vi "Barcode Scan State.vi"(1 "Barcode Scan Refnum":refnum<vi>, 2 "Stop Button Ref":refnum<vi>, 5 "Queue in":refnum<queue>, 9 "Test Results":T1, 11 "error in (no error)":errorcluster) -> (8 "Number of Buttons":u32=14, 10 "Test Results Out":T1, 15 "error out":errorcluster)   [LabVIEW 2016]
doc: "This VI performs the Wait for Barcode Scan State. It reads the config file in a while loop until a valid model number is read. Then determines hardware type, and updates UI based on hardware type."
uses:
  controls/Test Results.ctl
  C:/Program Files (x86)/National Instruments/LabVIEW 2016/examples/Design Patterns/Queued Message Handler/support/QMH Fundamentals - Message Cluster.ctl
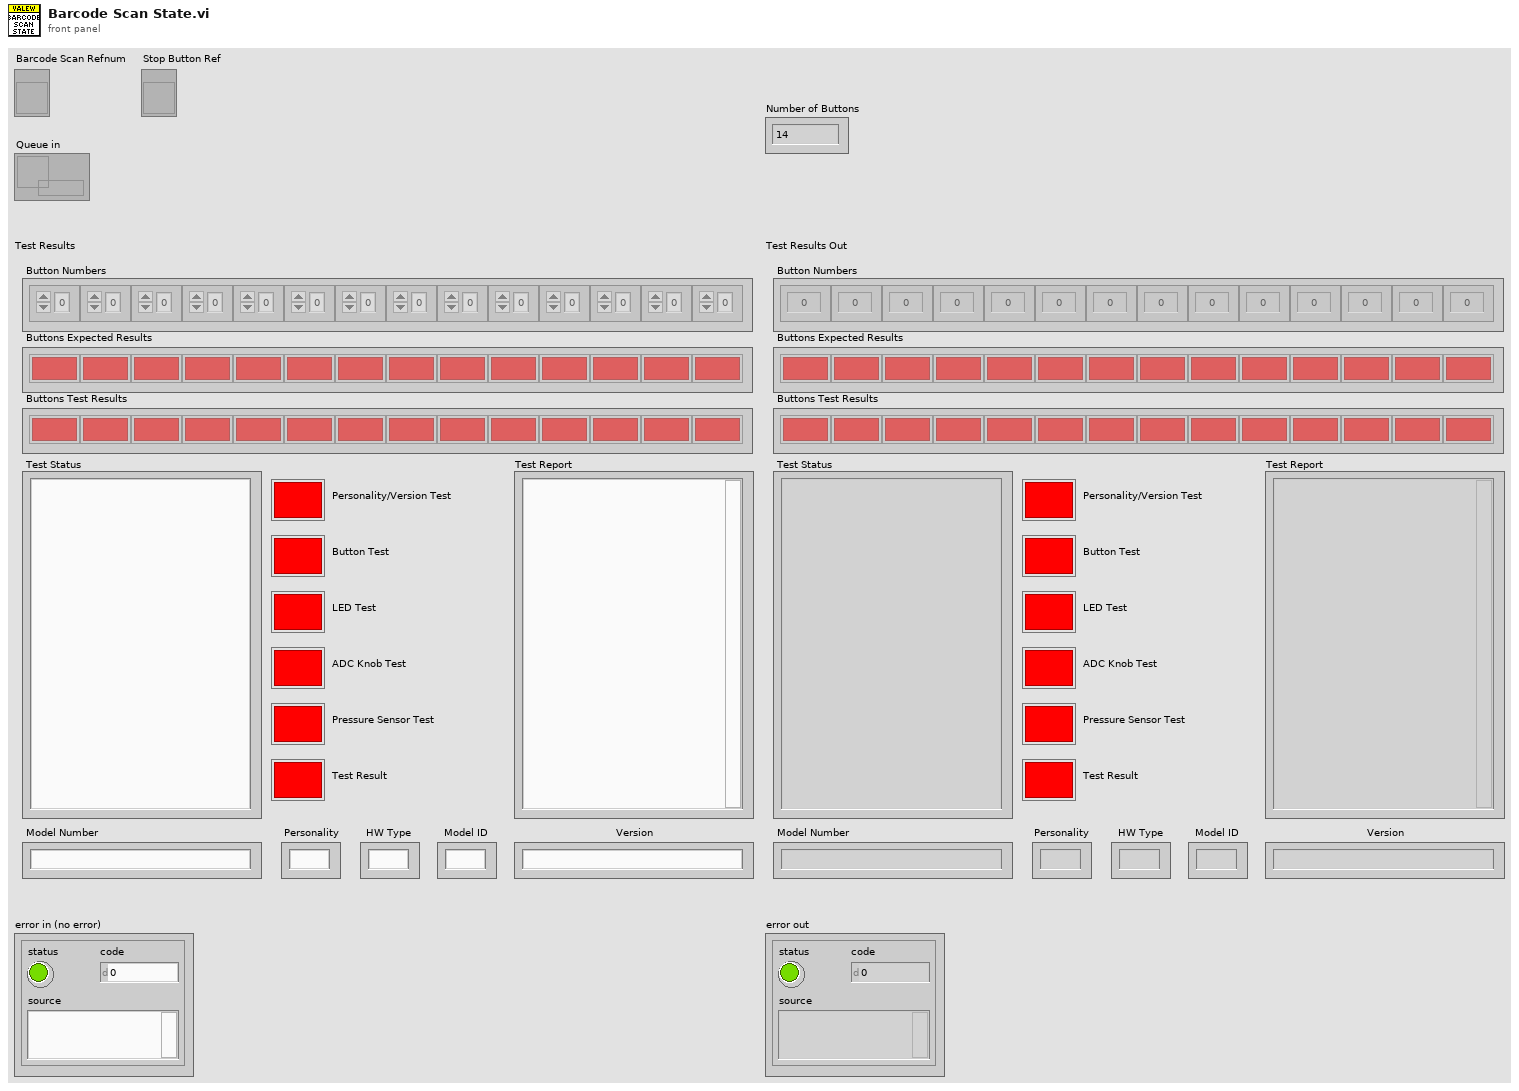
[diagram p1: front panel]
types:
  T1 = typedef "Test Results.ctl" = cluster{"Test Status":string, "Personality/Version Test ":bool, "Test Report":string, "Model Number":string, "Button Numbers":i32[], "Buttons Test Results":bool[], "Buttons Expected Results":bool[], "Model ID":string, "Personality":string, "HW Type":string, "Version":string, "Button Test":bool, "LED Test":bool, "ADC Knob Test":bool, "Pressure Sensor Test":bool, "Test Result":bool}
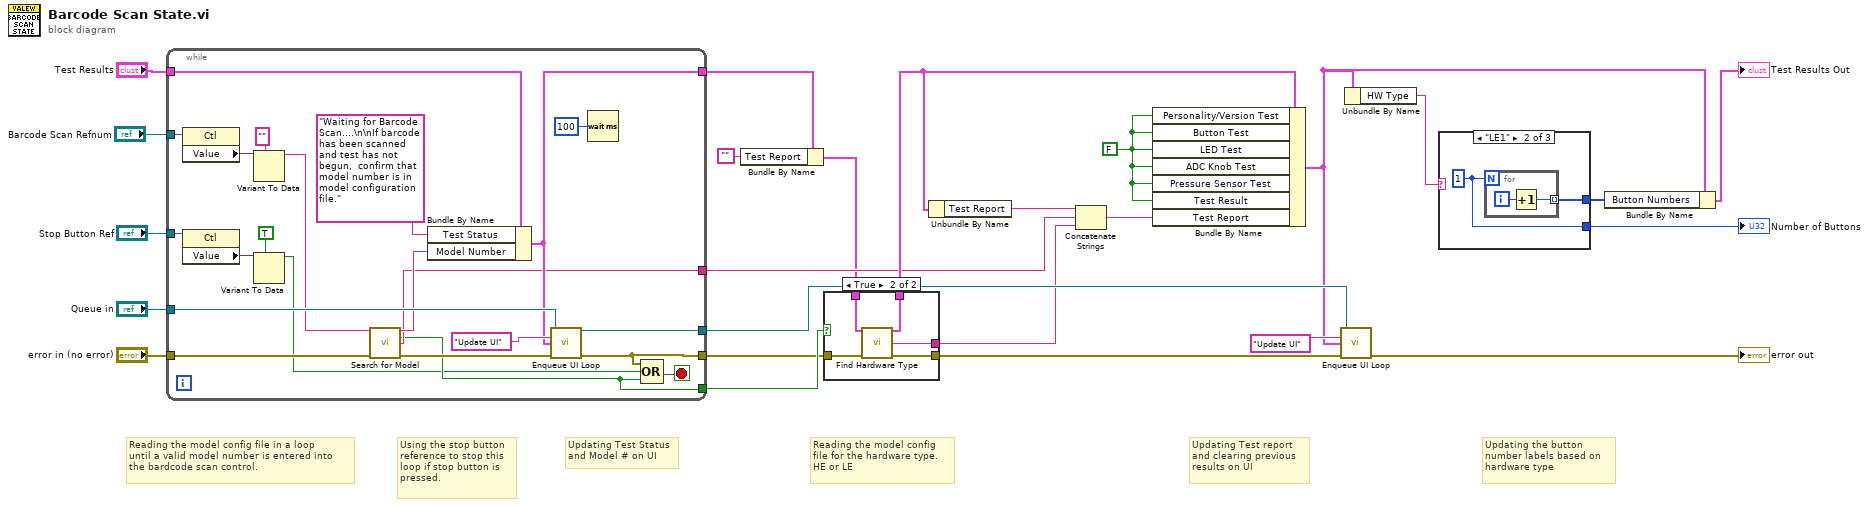
[diagram p0: block diagram]
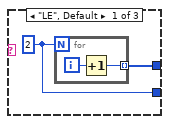
[diagram p2: hidden frame]
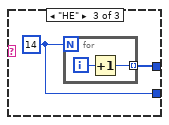
[diagram p3: hidden frame]
diagram:
  w1 = FALSE
  # "Updating Test Status\nand Model # on UI"
  # "Updating the button \nnumber labels based on \nhardware type"
  # "Updating Test report\nand clearing previous \nresults on UI"
  # "Reading the model config \nfile for the hardware type.\nHE or LE"
  # "Reading the model config file in a loop\nuntil a valid model number is entered into \nthe bardcode scan control."
  # "Using the stop button\nreference to stop this \nloop if stop button is\npressed."
  n1 = while {
    tunnel: "Test Results" -> [w44]
    tunnel: "error in (no error)" -> [w46]
    tunnel: "Queue in" -> [w41]
    tunnel: [w39] -> w5
    tunnel: [w35] -> w20
    tunnel: [w37] -> w22
    tunnel: [w36] -> w12
    tunnel: [w34] -> w25
    tunnel: "Barcode Scan Refnum" -> [w33]
    tunnel: "Stop Button Ref" -> [w28]
    stop <- w45 stop-if-true
    n2 = property class="Ctl"(reference=w33) -> ("Value"=w32:variant)  [unwired: 1 in, 2 out]
    n3 = property class="Ctl"(reference=w28) -> ("Value"=w29:variant)  [unwired: 1 in, 2 out]
    n4 = Variant To Data(type="", Variant=w32) -> (data=w31:string)  [unwired: 1 in, 1 out]
    n5 = Variant To Data(type=TRUE, Variant=w29) -> (data=w27:bool)  [unwired: 1 in, 1 out]
    n6 = call "Search for Model.vi"("Barcode Scan"=w31, "error in (no error)"=w46) -> ("Model Number"=w38:string, "Model Found?"=w34:bool, "Report Text"=w36:string, "error out"=w42:errorcluster)  [unwired: 10 in]
    n7 = Bundle By Name(cluster=w44, "Test Status"="Waiting for Barcode Scan....\n\nIf barcode has been scanned and test has not begun,  confirm that model number is in model configuration file.", "Model Number"=w38) -> (w39:T1)
    n8 = call "Enqueue UI Loop.vi"("UI Que In"=w41, "Message"="Update UI", "Test Results"=w39, "error in (no error)"=w42) -> ("UI Queue Out"=w37:refnum<queue>, "error out"=w35:errorcluster)  [unwired: 10 in]
    n9 = Wait (ms)(milliseconds to wait=u32 100) -> ()  [unwired: 1 out]
    n10 = Compound Arithmetic op=OR(w35, w27, w34) -> (w45:bool)
  }
  n11 = Bundle By Name(cluster=w5, "Test Report"="") -> (w4:T1)
  n12 = case shown="True" w25 {
    tunnel: w20 -> [w48 w54]
    tunnel: [w48 w53] -> w24
    tunnel: w4 -> [w49 w52]
    tunnel: [w49 w51] -> w13
    tunnel: [_ w50] -> w10
    frame False {
    }
    frame True {
      n13 = call "Find Hardware Type.vi"("Test Results In"=w52, "error in (no error)"=w54) -> ("Test Results Out"=w51:T1, "Report Text"=w50:string, "error out"=w53:errorcluster)  [unwired: 10 in, 1 out]
    }
  }
  n14 = Unbundle By Name(w13) -> ("Test Report"=w14:string)
  n15 = Concatenate Strings(w14, w12, w10) -> (w11:string)
  n16 = Bundle By Name(cluster=w13, "Personality/Version Test"=w1, "Button Test"=w1, "LED Test"=w1, "ADC Knob Test"=w1, "Pressure Sensor Test"=w1, "Test Result"=w1, "Test Report"=w11) -> (w8:T1)
  n17 = call "Enqueue UI Loop.vi"("UI Que In"=w22, "Message"="Update UI", "Test Results"=w8, "error in (no error)"=w24) -> ("error out"=→"error out":errorcluster)  [unwired: 10 in, 1 out]
  n18 = Unbundle By Name(w8) -> ("HW Type"=w9:string)
  n19 = case shown="\"LE1\"" w9 {
    tunnel: [w56 w60 w64] -> w7
    tunnel: [w55 w59 w63] -> w2
    frame "LE", Default {
      w55 = u32 2
      n20 = for {
        N: w55 -> [_]
        tunnel: [w57] -> w56 mode=indexing
        i -> [w58]
        n21 = Increment(x=w58) -> (x+1=w57:i32)
      }
    }
    frame "LE1" {
      w59 = u32 1
      n22 = for {
        N: w59 -> [_]
        tunnel: [w61] -> w60 mode=indexing
        i -> [w62]
        n23 = Increment(x=w62) -> (x+1=w61:i32)
      }
    }
    frame "HE" {
      w63 = 14
      n24 = for {
        N: w63 -> [_]
        tunnel: [w65] -> w64 mode=indexing
        i -> [w66]
        n25 = Increment(x=w66) -> (x+1=w65:i32)
      }
    }
  }
  "Number of Buttons" <- w2
  n26 = Bundle By Name(cluster=w8, "Button Numbers"=w7) -> (→"Test Results Out":T1)
